vi "Configure Measurement.vi"(8 "error in (no error)":errorcluster, 11 "Cap Bank Idot Measurement in":refnum<class "Cap Bank Idot Measurement.lvclass">) -> (0 "error out":errorcluster, 3 "Cap Bank Idot Measurement out":refnum<class "Cap Bank Idot Measurement.lvclass">)   [LabVIEW 2015, in "Cap Bank Idot Measurement.lvclass"]
uses:
  Cap Bank Idot Measurement.lvclass
  <vilib>/ActorFramework/Actor/Actor.lvclass/Actor.ctl
  Mag Lab Measure Controller Messages/Log Status Update Msg/Log Status Update Msg.lvclass/Log Status Update Msg.ctl
  <vilib>/ActorFramework/Message Enqueuer/Message Enqueuer.lvclass/Message Enqueuer.ctl
  <vilib>/ActorFramework/Message Enqueuer/Enqueue.vi
  <vilib>/ActorFramework/Message Priority Queue/Priority Enqueue.vi
  Mag Lab Measure Controller Messages/Log Status Update Msg/Log Status Update Msg.lvclass
  NI-DAQ/Mag Lab Measure/DAQmx Digitizer/DAQmx Digitizer.lvclass
  <vilib>/ActorFramework/Actor/Actor.lvclass
  Mag Lab Error Handler/Mag Lab Error Handler.lvclass
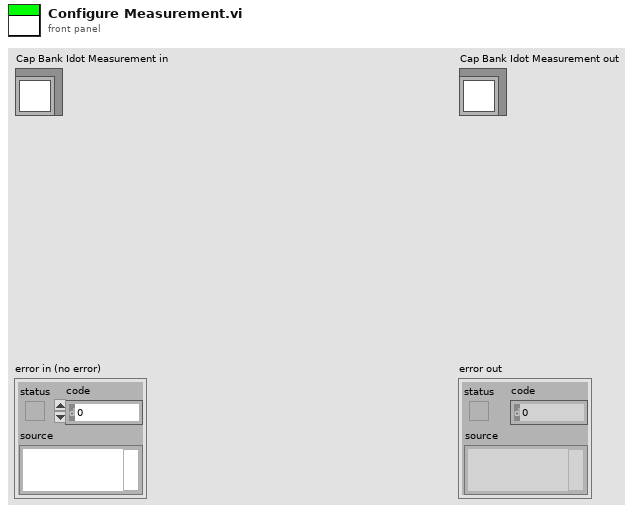
[diagram p1: front panel]
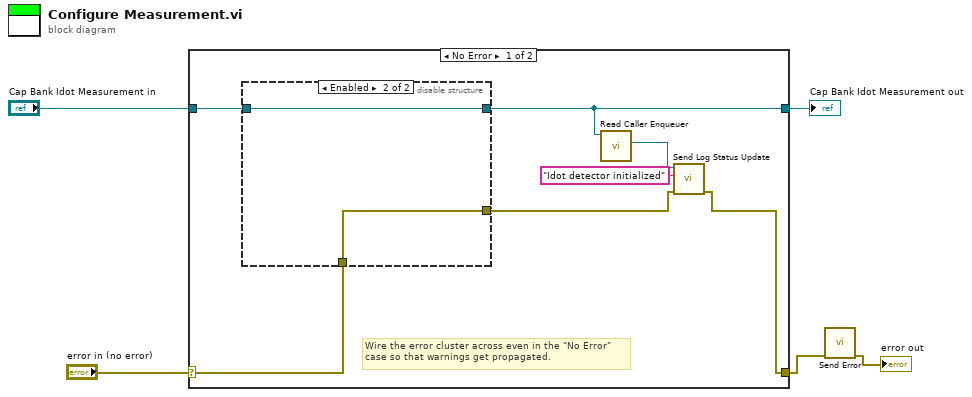
[diagram p0: block diagram]
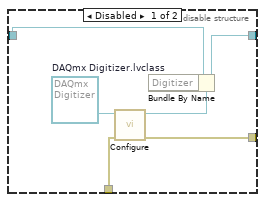
[diagram p2: hidden frame]
diagram:
  n1 = case shown="No Error" "error in (no error)" {
    selector: "error in (no error)" -> [w11 w22]
    tunnel: [w7 w22] -> w2
    tunnel: [w8 w21] -> w3
    tunnel: "Cap Bank Idot Measurement in" -> [w12 w21]
    frame No Error {
      # "Wire the error cluster across even in the \"No Error\"\ncase so that warnings get propagated."
      n2 = disable-structure shown="Enabled" {
        disable-tunnel: w12 -> [w18 w20]
        disable-tunnel: w11 -> [w15 w19]
        disable-tunnel: [w14 w20] -> w8
        disable-tunnel: [w13 w19] -> w6
        frame Disabled {
          w17 = refnum<class "DAQmx Digitizer.lvclass"> refnum  # DAQmx Digitizer.lvclass
          n3 = call-dynamic "Configure.vi"("error in (no error)"=w15, "DAQmx Digitizer in"=w17) -> ("error out"=w13:errorcluster, "DAQmx Digitizer out"=w16:refnum<class "DAQmx Digitizer.lvclass">)  [unwired: 8 in]
          n4 = Bundle By Name(cluster=w18, "Digitizer"=w16) -> (w14:refnum<class "Cap Bank Idot Measurement.lvclass">)
        }
        frame Enabled {
        }
      }
      n5 = call <vilib>:"Read Caller Enqueuer.vi"("Actor"=w8) -> ("Caller Enqueuer"=w9:refnum<class "Message Enqueuer.lvclass">)  [unwired: 10 in]
      n6 = call "Send Log Status Update.vi"("error in (no error)"=w6, "Status"="Idot detector initialized", "Message Enqueuer"=w9) -> ("error out"=w7:errorcluster)  [unwired: 7 in, 1 out]
    }
    frame Error {
    }
  }
  "Cap Bank Idot Measurement out" <- w3
  n7 = call "Send Error.vi"("error in (no error)"=w2) -> ("error out"=→"error out":errorcluster)  [unwired: 9 in, 1 out]
